vi "StartProcesses.vi"(8 "error in (no error)":errorcluster, 11 "JKI SMO in":refnum<class "JKI SMO.lvclass">) -> (0 "error out":errorcluster, 3 "JKI SMO out":refnum<class "JKI SMO.lvclass">)   [LabVIEW 2013, in "JKI SMO.lvclass"]
doc: "Starts all processes in the JKI SMO.\n\n---------------------------------------------------------------\nJKI State Machine Objects™\nhttp://jki.net/state-machine-objects/\nCopyright (C) 2005-2015, JKI <info@jki.net>\nALL RIGHTS RESERVED"
uses:
  JKI SMO.lvclass
  JKI SMO.lvclass/JKI SMO.ctl
panel:
  in  "ms timeout (-1)":i32=-1
  # "For instructions on how to use the JKI State Machine Objects, examples and video tutorials, visit:\nhttp://jki.net/state-machine-objects/\n\nJKI State Machine Objects™\nhttp://jki.net/state-machine-objects/\nCopyright (C) 2005-2015, JKI <info@jki.net>\nALL RIGHTS RESERVED"
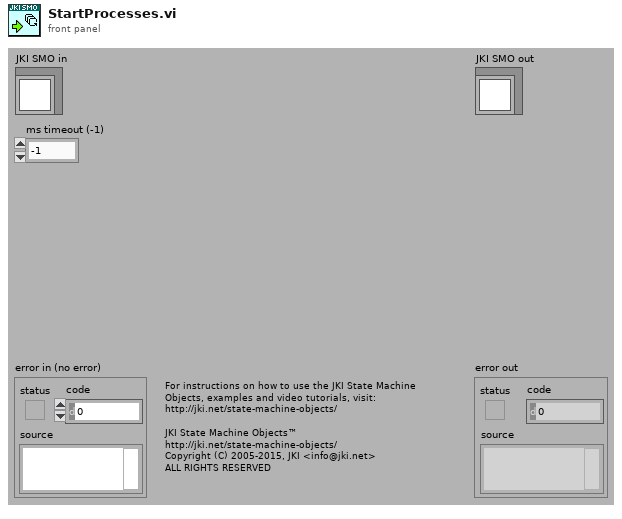
[diagram p1: front panel]
types:
  T1 = typedef "JKI SMO.lvclass/RegisteredProcessData--Cluster.ctl" = cluster{"Name":string, "Static VI Ref":refnum<vi>}
  T2 = typedef "pSubSystem.lvclass/pSubSystem.PrivateData--Cluster.ctl" = cluster{"Processes Clone VI Ref [ ]":refnum<vi>[], "Processes Clone Name [ ]":string[], "Process Sync RendezVous":T3, "Protected Events":T4}
  T3 = typedef "Rendezvous RefNum" = refnum<k1>
  T4 = typedef "pSubSystem.lvclass/pSubSystem.ProtectedEvents--Cluster.ctl" = cluster{"StopProcesses":refnum<user-event>, "AbortProcesses":refnum<user-event>}
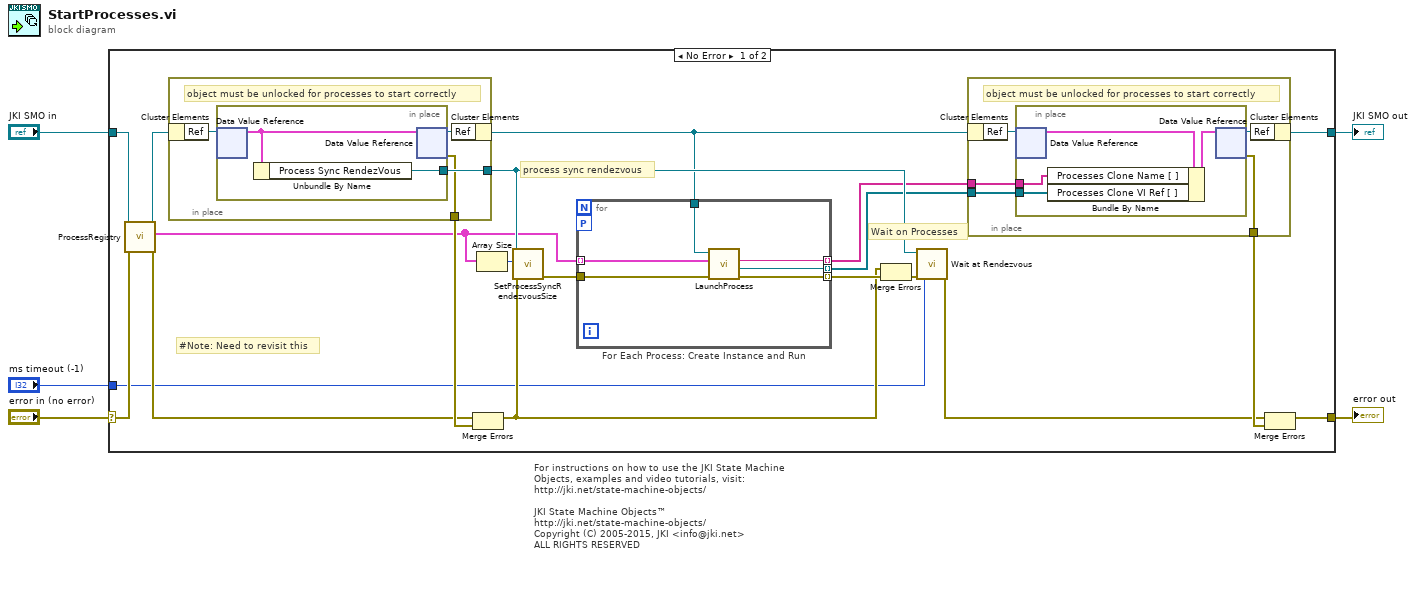
[diagram p0: block diagram]
diagram:
  # "For instructions on how to use the JKI State Machine Objects, examples and video tutorials, visit:\nhttp://jki.net/state-machine-objects/\n\nJKI State Machine Objects™\nhttp://jki.net/state-machine-objects/\nCopyright (C) 2005-2015, JKI <info@jki.net>\nALL RIGHTS RESERVED"
  n1 = case shown="No Error" "error in (no error)" {
    selector: "error in (no error)" -> [w15 w48]
    tunnel: [w8 w48] -> w4
    tunnel: [w12 w47] -> w2
    tunnel: "JKI SMO in" -> [w18 w47]
    tunnel: "ms timeout (-1)" -> [w6 _]
    frame No Error {
      # "#Note: Need to revisit this"
      # "process sync rendezvous"
      # "Wait on Processes"
      n2 = call-dynamic "ProcessRegistry.vi"("error in (no error)"=w15, "JKI SMO in"=w18) -> ("error out"=w14:errorcluster, "Registered Process [ ]"=w16:T1[], "JKI SMO out"=w17:refnum<class "JKI SMO.lvclass">)  [unwired: 7 in]
      n3 = in-place {
        in-place-border: [w38] -> w23
        in-place-border: [w37] -> w20
        # "object must be unlocked for processes to start correctly"
        n4 = in-place-cluster #1(w17) -> ("Ref"=w36:refnum<data-value>)
        n5 = in-place {
          in-place-border: [w40] -> w38
          n6 = in-place-dvr #2(w36) -> (w39:T2)  [unwired: 1 out]
          n7 = Unbundle By Name(w39) -> ("Process Sync RendezVous"=w40:T3)
          n8 = in-place-dvr #2(w39) -> (w35:refnum<data-value>, w37:errorcluster)
        }
        n9 = in-place-cluster #1("Ref"=w35) -> (w13:refnum<class "JKI SMO.lvclass">)
      }
      n10 = Merge Errors(w14, w20) -> (w19:errorcluster)
      n11 = Array Size(array=w16) -> (size(s)=w24:i32)
      n12 = call "SetProcessSyncRendezvousSize.vi"("error in"=w19, "# processes"=w24, "Process Sync Rendezvous"=w23) -> ("error out"=w25:errorcluster)  [unwired: 8 out]
      n13 = for "For Each Process: Create Instance and Run" {
        tunnel: w16 -> [w45] mode=indexing
        tunnel: w13 -> [w44]
        tunnel: w25 -> [w46]
        tunnel: [w43] -> w22 mode=indexing
        workers-P: _ -> [_]
        tunnel: [w42] -> w11 mode=indexing
        tunnel: [w41] -> w7 mode=indexing
        n14 = call "LaunchProcess.vi"("error in (no error)"=w46, "Process Data"=w45, "JKI SMO in"=w44) -> ("error out"=w43:errorcluster, "VI Ref Out"=w42:refnum<vi>, "Name"=w41:string)  [unwired: 5 in, 1 out]
      }
      n15 = Merge Errors(w19, w22) -> (w21:errorcluster)
      n16 = call <vilib>:"Wait at Rendezvous.vi"("error in (no error)"=w21, "ms timeout (-1)"=w6, "rendezvous"=w23) -> ("error out"=w9:errorcluster)  [unwired: 4 out]
      n17 = in-place {
        in-place-border: [w30] -> w10
        in-place-border: w11 -> [w27]
        in-place-border: w7 -> [w26]
        # "object must be unlocked for processes to start correctly"
        n18 = in-place-cluster #3(w13) -> ("Ref"=w29:refnum<data-value>)
        n19 = in-place {
          in-place-border: w27 -> [w32]
          in-place-border: w26 -> [w31]
          n20 = in-place-dvr #4(w29) -> (w34:T2)  [unwired: 1 out]
          n21 = Bundle By Name(cluster=w34, "Processes Clone Name [ ]"=w31, "Processes Clone VI Ref [ ]"=w32) -> (w33:T2)
          n22 = in-place-dvr #4(w33) -> (w28:refnum<data-value>, w30:errorcluster)
        }
        n23 = in-place-cluster #3("Ref"=w28) -> (w12:refnum<class "JKI SMO.lvclass">)
      }
      n24 = Merge Errors(w9, w10) -> (w8:errorcluster)
    }
    frame Error {
    }
  }
  "error out" <- w4
  "JKI SMO out" <- w2
